vi "import ODB.vi"(0 "Dongle Fitted event Refnum in":T2, 2 "Programming Data":T4, 3 "APG Config":T3={"IPF Folder"=path "", "Results Folder"=path "", "Trace Folder"=path "", "a3DiCAD"={"Plot Spacing"=0.0, "TCF"=enum."STANDARD", "LeadLimit"=0, "a3DiCADDebug"=FALSE, "ODB"={"PrimePartNumber"=[], "SecondPartNumber"=[], "Height"={"PRP_CMP"="", "HEIGHT"=""}, "Units"={"PRP_CMP"="", "UNITS"=""}}, "PasteHeight"=0.0, "Inspection Performance"=TRUE}, "a3DiCADcfg"=path "", "Board Library"={"Board Library file"=path "", "Board library model folder"=path "", "Not Fittted/Fitted Components"=path "", "Panel Picture File"=path "", "Components"=enum."Fitted"}, "Site Library"={"Site Library file"=path "", "Site library model folder"=path ""}, "System Library"={"System Library file"=path "", "System library model folder"=path ""}, "ODB++ file"=path "", "Side ID Alias"={"Top"="", "Bottom"=""}}, 4 "Data":T10, 5 "error in":errorcluster, 6 "Edit VI":refnum<vi>, 7 "FP ctrl references":T1) -> (14 "Programming Data out":T4, 16 "Data out":T10, 17 "Dongle fitted":bool, 18 "APG Config":T3={"IPF Folder"=path "", "Results Folder"=path "", "Trace Folder"=path "", "a3DiCAD"={"Plot Spacing"=0.0, "TCF"=enum."STANDARD", "LeadLimit"=0, "a3DiCADDebug"=FALSE, "ODB"={"PrimePartNumber"=[], "SecondPartNumber"=[], "Height"={"PRP_CMP"="", "HEIGHT"=""}, "Units"={"PRP_CMP"="", "UNITS"=""}}, "PasteHeight"=0.0, "Inspection Performance"=TRUE}, "a3DiCADcfg"=path "", "Board Library"={"Board Library file"=path "", "Board library model folder"=path "", "Not Fittted/Fitted Components"=path "", "Panel Picture File"=path "", "Components"=enum."Fitted"}, "Site Library"={"Site Library file"=path "", "Site library model folder"=path ""}, "System Library"={"System Library file"=path "", "System library model folder"=path ""}, "ODB++ file"=path "", "Side ID Alias"={"Top"="", "Bottom"=""}}, 19 "error out":errorcluster)   [LabVIEW 2013, in "Manipulate IPF.lvlib"]
uses:
  Manipulate IPF.lvlib
  type_def/files.ctl
  3013/code/Modules/Inspection/Data/Panel_class/type_def/Config File data.ctl
  3013/code/Modules/Inspection/type_def/Pos and Rot.ctl
  3013/code/Modules/Inspection/Data/PCB_class/type_def/PCB Params.ctl
  3013/code/Modules/Inspection/Data/Panel_class/type_def/BarCode Params.ctl
  3013/code/Modules/Barcode Reader/type_def/id.ctl
  Settings/type_def/APG Config.ctl
  3013/code/Modules/GUI/GUI_5/subPanels/edit/type_def/data.ctl
  3013/code/Modules/Configuration/type_def/Scan Params.ctl
  3013/code/Modules/Configuration/type_def/Profile Resolution.ctl
  3013/code/Modules/Preprocess Data/type_def/direction.ctl
  3013/code/Modules/Inspection/Data/Panel_class/type_def/inspection data.ctl
  3013/code/Modules/Inspection/type_def/Range Limits.ctl
  type_def/Dongle fitted event refnum.ctl
  type_def/Import ODB state.ctl
  3013/code/Modules/Scanner/Robot/type_def/robot scan params DBL.ctl
  3013/code/Modules/Scanner/Robot/type_def/point DBL.ctl
  type_def/Picture FGV commands.ctl
  Pack Data/type_def/file types.ctl
  type_def/IPF cmd.ctl
  <userlib>/_OpenG.lib/file/file.llb/File Exists - Scalar__ogtk.vi
  <userlib>/_OpenG.lib/file/file.llb/Convert File Extension (Path)__ogtk.vi
  <vilib>/Utility/cursorutil.llb/Set Cursor (Icon Pict).vi
  Settings/Globals/apg_cfg_global.vi
  Conversion/conversion.lvlib
  3013/code/Modules/Configuration/Config.lvlib
  3013/code/Modules/Barcode Reader/Barcode Reader.lvlib
  3013/code/Modules/Inspection/Data/Panel_class/Panel.lvclass
  3013/code/Modules/Inspection/Inspection.lvlib
  3013/code/Modules/Inspection/Data/PCB_class/PCB.lvclass
  3013/code/Modules/Preprocess Data/PreProcess.lvlib
  3013/code/Modules/Scanner/Robot/Robot.lvlib
  3013/code/Modules/GUI/GUI_5/subPanels/edit/edit.lvlib
  Pack Data/Pack Files.lvlib
  Update TCF/TCF update.lvlib
  a3Di APG.lvlib
  Settings/APG_settings.lvlib
  Mike/APG_mike a3Di.lvlib
  Gerber import/Gerber import.lvlib
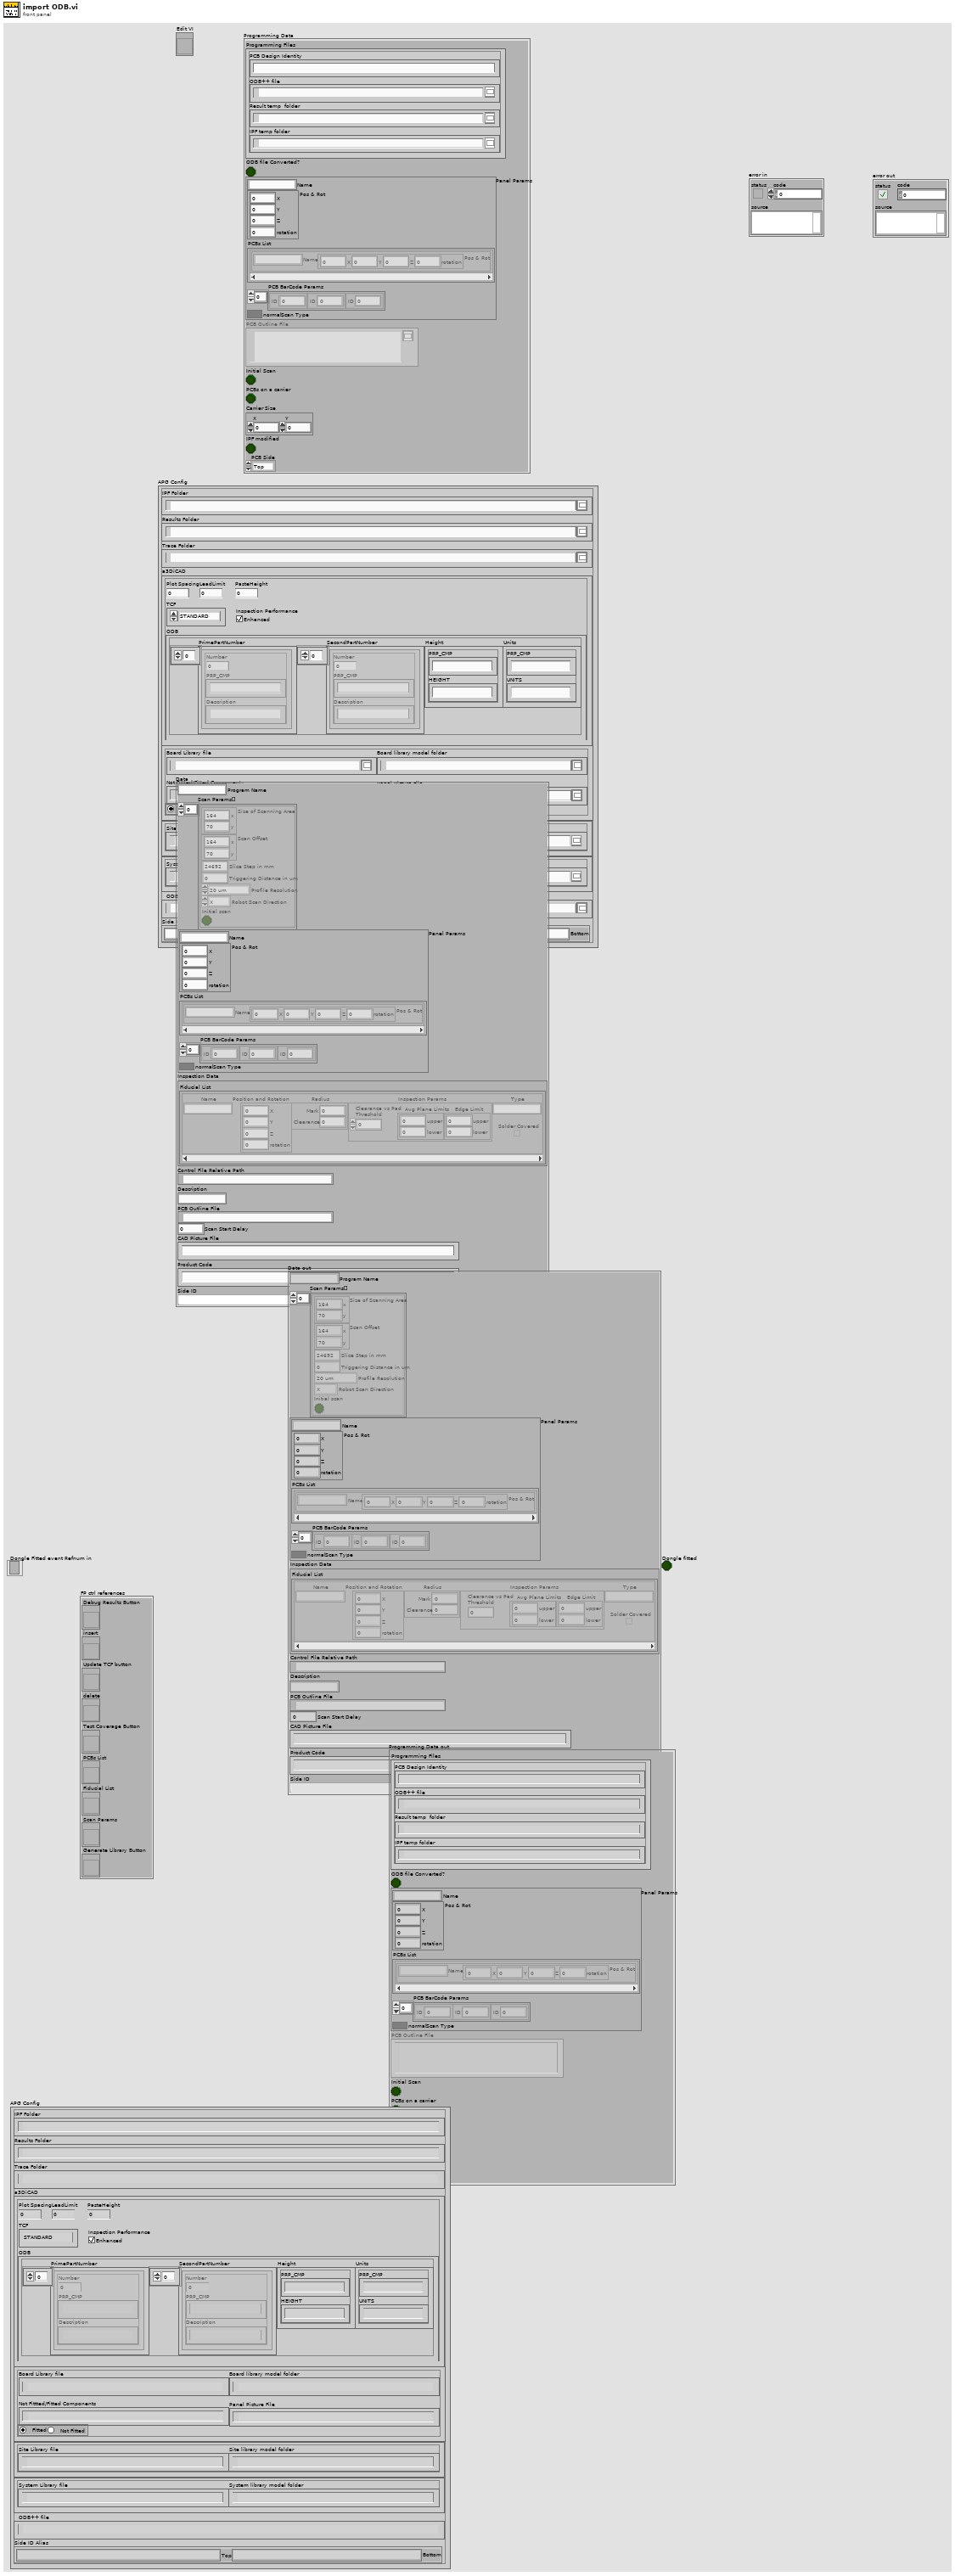
[diagram p1: front panel]
types:
  T1 = cluster{"Debug Results Button":refnum<vi>, "insert":refnum<vi>, "Update TCF button":refnum<vi>, "delete":refnum<vi>, "Test Coverage Button":refnum<vi>, "PCBs List":refnum<vi>, "Fiducial List":refnum<vi>, "Scan Params":refnum<vi>, "Generate Library Button":refnum<vi>}
  T2 = typedef "Dongle fitted event refnum.ctl" = refnum<event-registration>
  T3 = typedef "APG_settings.lvlib/APG Config.ctl" = cluster{"IPF Folder":path, "Results Folder":path, "Trace Folder":path, "a3DiCAD":cluster{"Plot Spacing":dbl, "TCF":enum16{"STANDARD", "PASTE", "LEAD"}, "LeadLimit":u32, "a3DiCADDebug":bool, "ODB":cluster{"PrimePartNumber":cluster{"Number":u32, "PRP_CMP":string, "Description":string}[], "SecondPartNumber":cluster{"Number":u32, "PRP_CMP":string, "Description":string}[], "Height":cluster{"PRP_CMP":string, "HEIGHT":string}, "Units":cluster{"PRP_CMP":string, "UNITS":string}}, "PasteHeight":dbl, "Inspection Performance":bool}, "a3DiCADcfg":path, "Board Library":cluster{"Board Library file":path, "Board library model folder":path, "Not Fittted/Fitted Components":path, "Panel Picture File":path, "Components":enum32{"Fitted", "Not Fitted "}}, "Site Library":cluster{"Site Library file":path, "Site library model folder":path}, "System Library":cluster{"System Library file":path, "System library model folder":path}, "ODB++ file":path, "Side ID Alias":cluster{"Top":string, "Bottom":string}}
  T4 = typedef "a3Di APG.lvlib/files.ctl" = cluster{"Programming Files":cluster{"PCB Design Identity":string, "ODB++ file":path, "Result temp  folder":path, "IPF temp folder":path}, "ODB file Converted?":bool, "Panel Params":T5, "PCB Outline File":path, "Initial Scan":bool, "PCBs on a carrier":bool, "Carrier Size":cluster{"X":dbl, "Y":dbl}, "IPF modified":bool, "PCB Side":enum16{"Top", "Bottom"}}
  T5 = typedef "Inspection.lvlib/Panel.lvclass/Config File data.ctl" = cluster{"Name":string, "Pos & Rot":T6, "PCBs List":cluster{"PCB Params":T7}[], "PCB BarCode Params":T8[], "Scan Type":bool}
  T6 = typedef "Inspection.lvlib/Pos and Rot.ctl" = cluster{"X":dbl, "Y":dbl, "Z":dbl, "rotation":dbl}
  T7 = typedef "Inspection.lvlib/PCB.lvclass/PCB Params.ctl" = cluster{"Name":string, "Pos & Rot":T6}
  T8 = typedef "Inspection.lvlib/Panel.lvclass/BarCode Params.ctl" = cluster{"ID":T9}
  T9 = typedef "Barcode Reader.lvlib/id.ctl" = u8
  T10 = typedef "GUI.lvlib/subPanel.lvlib/edit.lvlib/data.ctl" = cluster{"Program Name":string, "Scan Params[]":T11[], "Panel Params":T5, "Inspection Data":T14, "Control File Relative Path":path, "Description":string, "PCB Outline File":path, "Scan Start Delay":dbl, "CAD Picture File":string, "Product Code":string, "Side ID":string}
  T11 = typedef "Config.lvlib/Scan Params.ctl" = cluster{"Size of Scanning Area":cluster{"x":dbl, "y":dbl}, "Scan Offset":cluster{"x":dbl, "y":dbl}, "Slice Step in mm":dbl, "Triggering Distance in mm":dbl, "Triggering Distance in um":dbl, "Profile Resolution":T12, "Version":string, "Robot Scan Direction":T13, "Initial scan":bool}
  T12 = typedef "Config.lvlib/Profile Resolution.ctl" = enum8{"20 um", "40 um"}
  T13 = typedef "PreProcess.lvlib/direction.ctl" = enum8{"X", "Y"}
  T14 = typedef "Inspection.lvlib/Panel.lvclass/inspection data.ctl" = cluster{"Fiducial List":cluster{"Name":string, "Position and Rotation":T6, "Radius":cluster{"Mark":dbl, "Clearance":dbl}, "Inspection Params":cluster{"Clearance vs Pad\nThreshold":dbl, "Avg Plane Limits":T15, "Edge Limit":T15}, "Type":string, "Solder Covered":bool}[]}
  T15 = typedef "Inspection.lvlib/Range Limits.ctl" = cluster{"upper":sgl, "lower":sgl}
  T16 = typedef "Manipulate IPF.lvlib/Import ODB state.ctl" = enum16{"Select format", "Select ODB++", "Extract ODB++", "Extract Gerber", "Select PCBs", "Scan area", "Select Fiducials", "Update TCF, save Files", "Cancel", "Exit", "Update CAD Picture"}
  T17 = typedef "Robot.lvlib/robot scan params DBL.ctl" = cluster{"Zero":T18, "Zero Speed":T18, "Distance":T18, "Speed":T18, "# of Slices":dbl, "Trigg Distance":dbl, "Robot Scan Direction":T13, "Next":cluster{"Next Zero":T18, "Next Robot Scan Direction":T13}}
  T18 = typedef "Robot.lvlib/point DBL.ctl" = cluster{"X":dbl, "Y":dbl}
  T19 = cluster{"Programming Files":cluster{"PCB Design Identity":string, "ODB++ file":path, "Result  folder":path, "Tar file":path}, "ODB file Converted?":bool, "Inspection Setup Data":cluster{"Inspection Program  file ":path, "PCB Scanning Area":cluster{"X":dbl, " Y":dbl}, "PCB Offset":cluster{" X":dbl, " Y":dbl}, "Scanning area  bot left and top right":cluster{"X":dbl, "Y":dbl}[], "Fiducials from scan":cluster{"Fiducial Name":string, "Fiducial co-ordinate":cluster{"X":dbl, "Y":dbl}}[], "TCF  file ":path, "Robot Scan Params DBL":T17, "Scan offset adjustment":cluster{"X":dbl, " Y":dbl}}, "Panel Params":T5, "PCB Outline File":path, "Inspection setup completed":bool, "PCB Layer scanned":enum16{"Bottom PCB Layer", "Top PCB Layer"}, "PCBs on a carrier":bool, "Carrier Size":cluster{"X":dbl, "Y":dbl}}
  T20 = typedef "Manipulate IPF.lvlib/Picture FGV commands.ctl" = enum16{"No Action", "Set Update Picture", "Set Delete Picture", "Get Picture action"}
  T21 = typedef "Pack Files.lvlib/file types.ctl" = enum16{"ODB", "TCF", "CAD Outline", "Config", "Inspection Prog", "a3Di-bin", "Results", "CAD Labels", "CAD Pads", "calScan_fid", "calScan_cal-tab", "PCB_SerialNumber", "CAD_Assembly", "Version", "Old Results", "CAD Picture", "Old TCF"}
  T22 = typedef "Manipulate IPF.lvlib/IPF cmd.ctl" = enum16{"New IPF", "Edit IPF", "Copy IPF", "Rename IPF", "Delete IPF", "Reload IPF", "Load all IPF"}
  T23 = enum16{"Left Button", "Center Button", "Right Button", "Window Close"}
  T24 = typedef "GUI.lvlib/subPanel.lvlib/edit.lvlib/GUI Panel & PCB params.ctl" = cluster{"Panel Params":T25, "PCBs List":T26}
  T25 = typedef "GUI.lvlib/subPanel.lvlib/edit.lvlib/GUI Panel Params.ctl" = cluster{"Name":string, "Pos & Rot":T6}
  T26 = typedef "GUI.lvlib/subPanel.lvlib/edit.lvlib/GUI PCB List.ctl" = cluster{"PCB Params":T7, "Barcode\nReader":cluster{"ID":T9}, "insert":bool, "delete":bool}[]
  T27 = cluster{"Scanning Area X in mm":dbl, "Scanning Area Y in mm":dbl}
  T28 = typedef "GUI.lvlib/subPanel.lvlib/edit.lvlib/GUI Fiducial List.ctl" = cluster{"Fiducial":cluster{"Name":string, "Pos & Rot":T6, "Radius":cluster{"Mark":dbl, "Clearance":dbl}, "Inspection Params":cluster{"Clearance vs\nPad Threshold":dbl, "Avg Plane Limits":T15, "Edge Limit":T15}, "Type":string, "Solder Covered":bool}, "insert":bool, "delete":bool}[]
  T29 = enum8{"Enabled", "Disabled", "Disabled and Grayed Out"}
  T30 = cluster{"APG":cluster{"APG SIN":string, "APG version":string}, "Installed Programs":cluster{"task name":string, "task version":string}[]}
  T31 = cluster{"task name":string, "task version":string}[]
  T32 = cluster{"Program":enum16{"APG", "Inspection Station"}, "APG":cluster{"APG SIN":string, "APG version":string}, "Installed Programs":cluster{"task name":string, "task version":string}[]}
  T33 = typedef "Manipulate IPF.lvlib/Picture FGV actions.ctl" = enum16{"No Action", "Update Picture", "Delete Picture"}
  T34 = cluster{"Name":string, "Position and Rotation":T6, "Radius":cluster{"Mark":dbl, "Clearance":dbl}, "Inspection Params":cluster{"Clearance vs Pad\nThreshold":dbl, "Avg Plane Limits":T15, "Edge Limit":T15}, "Type":string, "Solder Covered":bool}[]
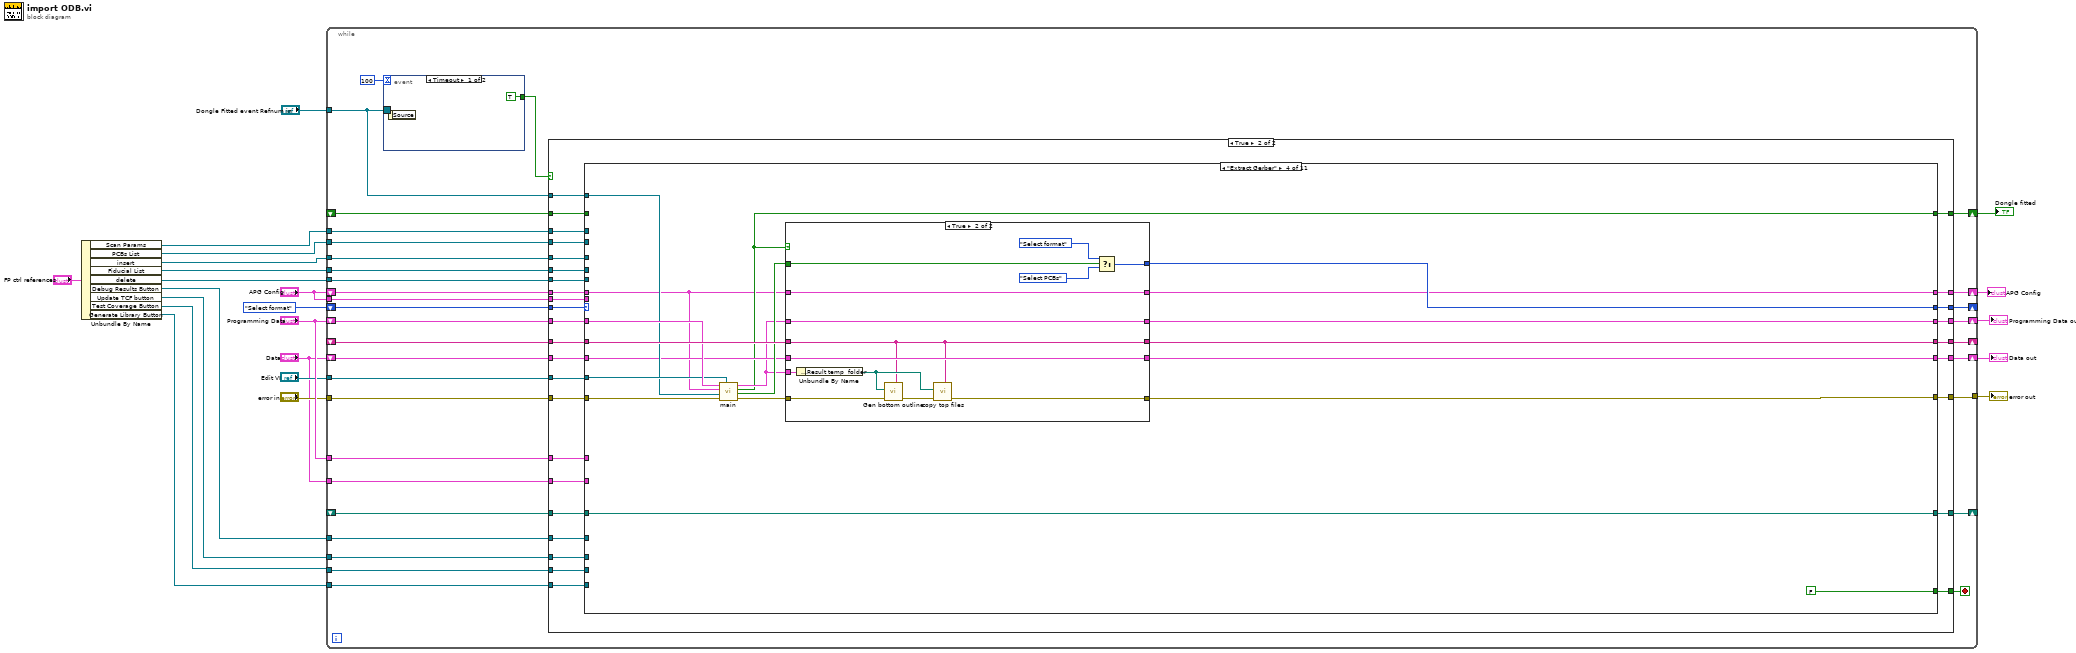
[diagram p0: block diagram]
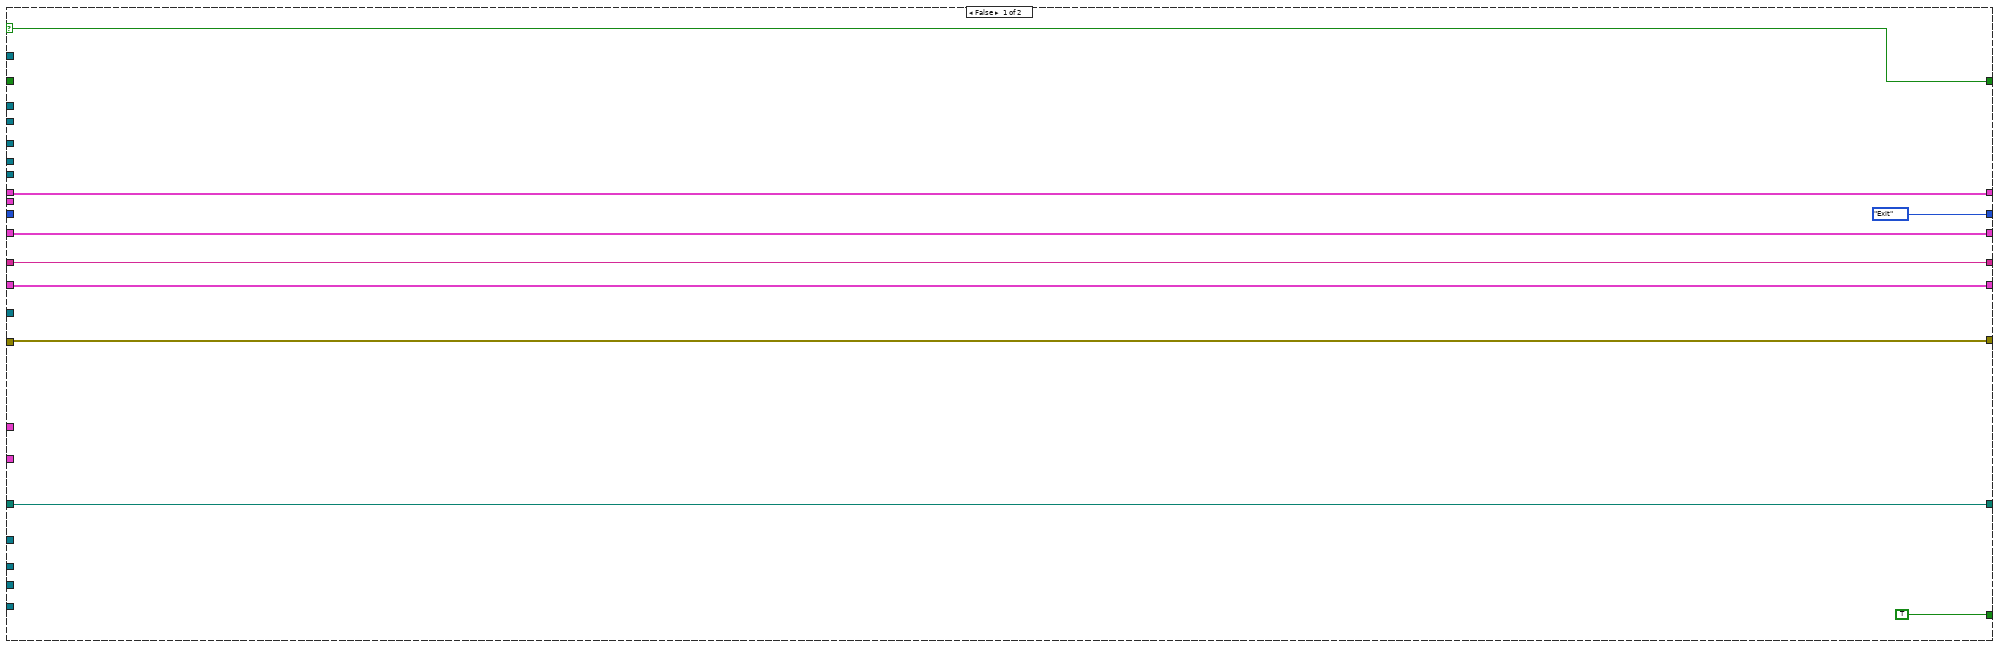
[diagram p2: hidden frame]
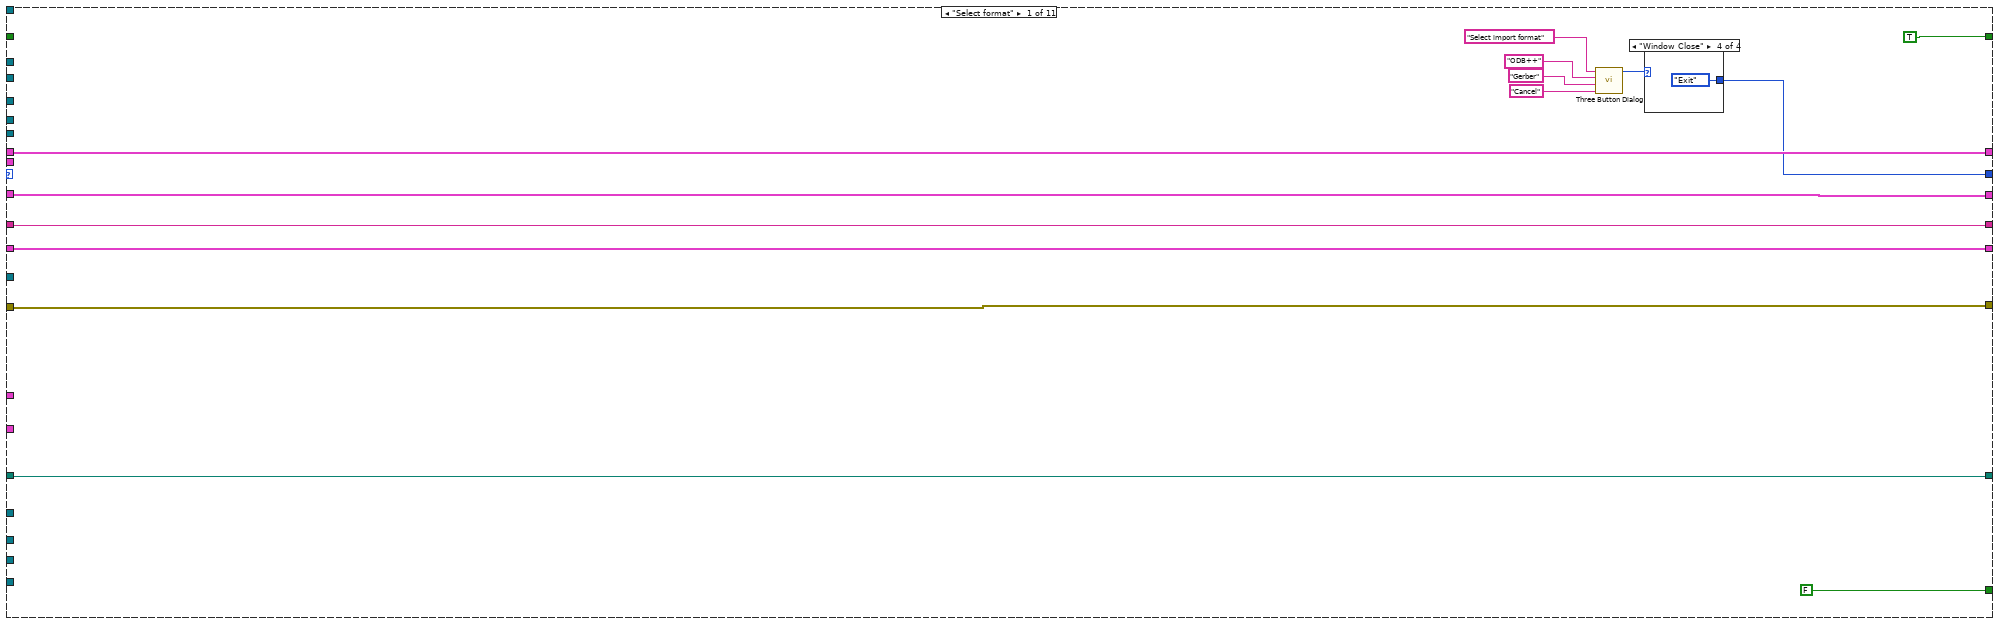
[diagram p3: hidden frame]
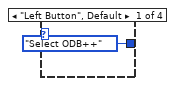
[diagram p4: hidden frame]
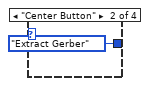
[diagram p5: hidden frame]
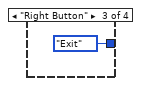
[diagram p6: hidden frame]
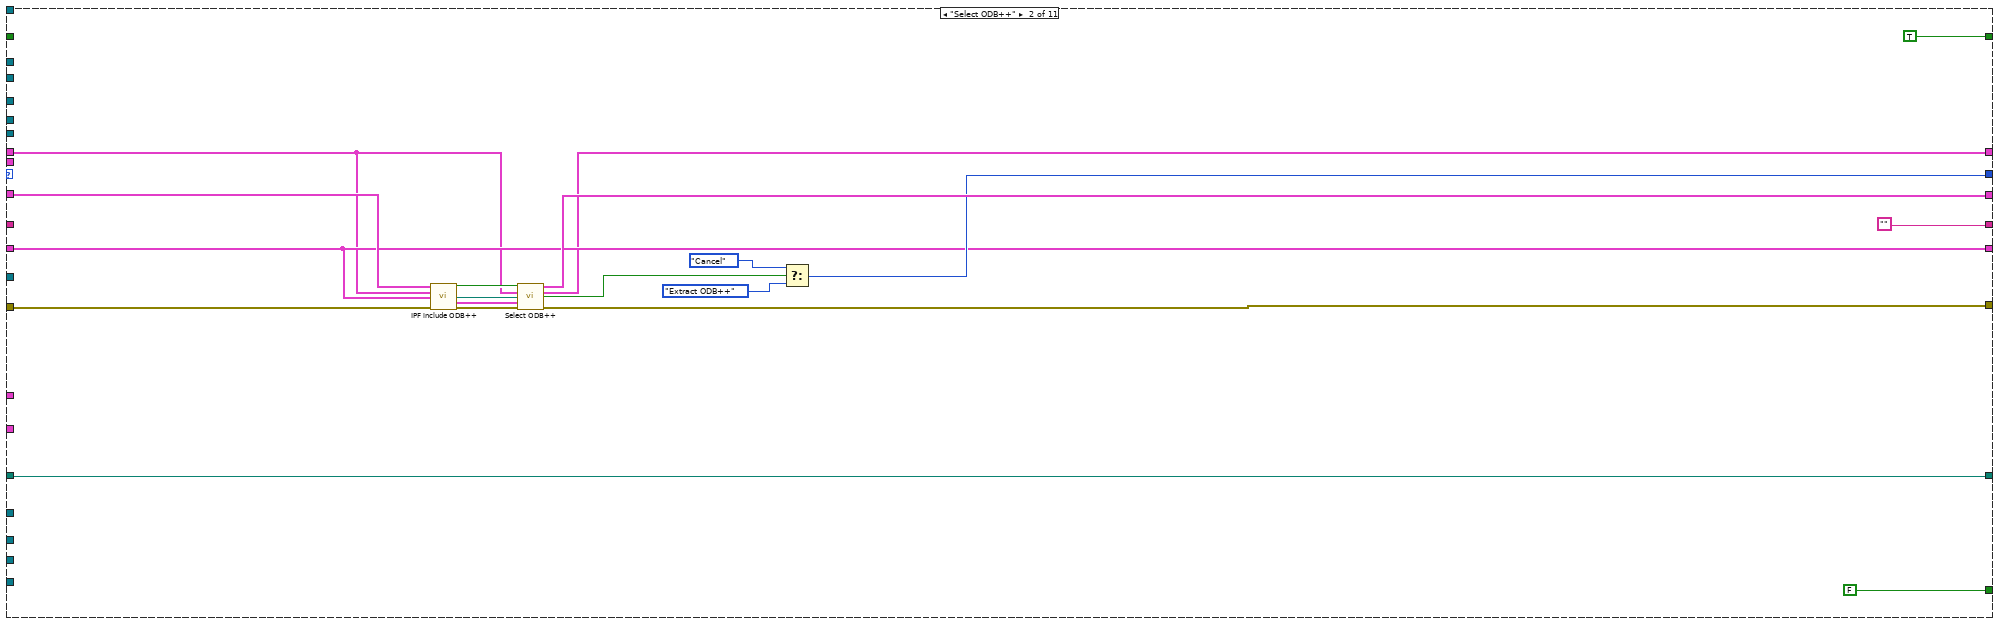
[diagram p7: hidden frame]
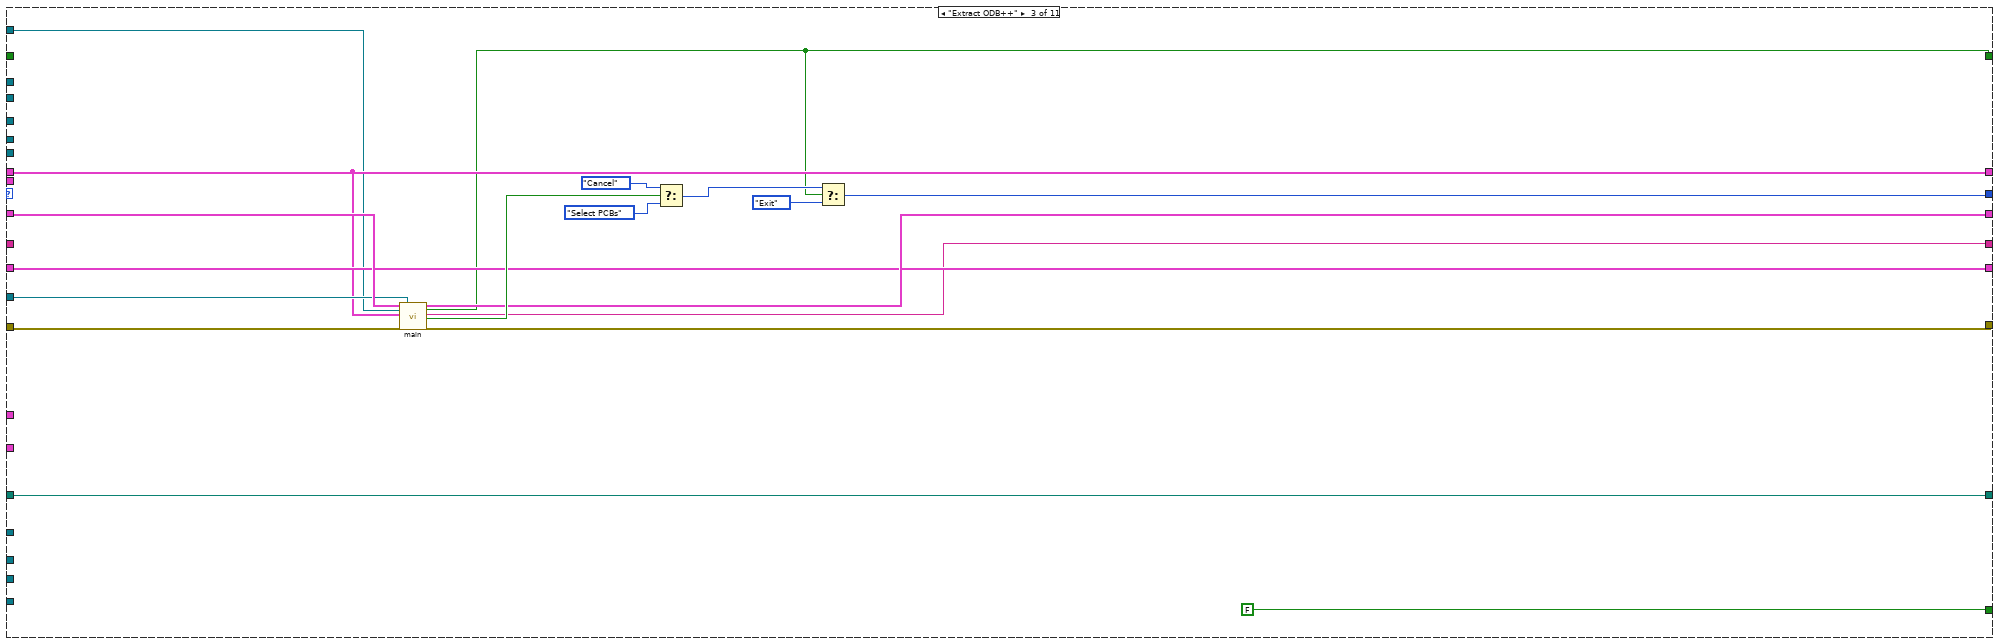
[diagram p8: hidden frame]
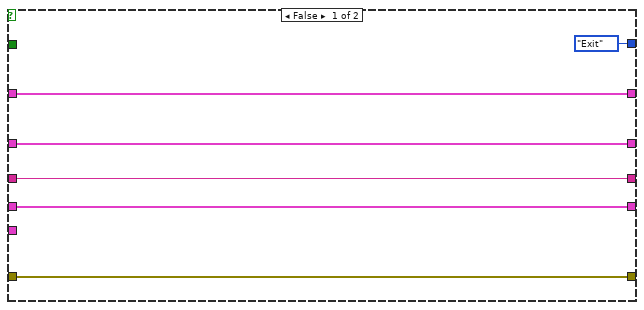
[diagram p9: hidden frame]
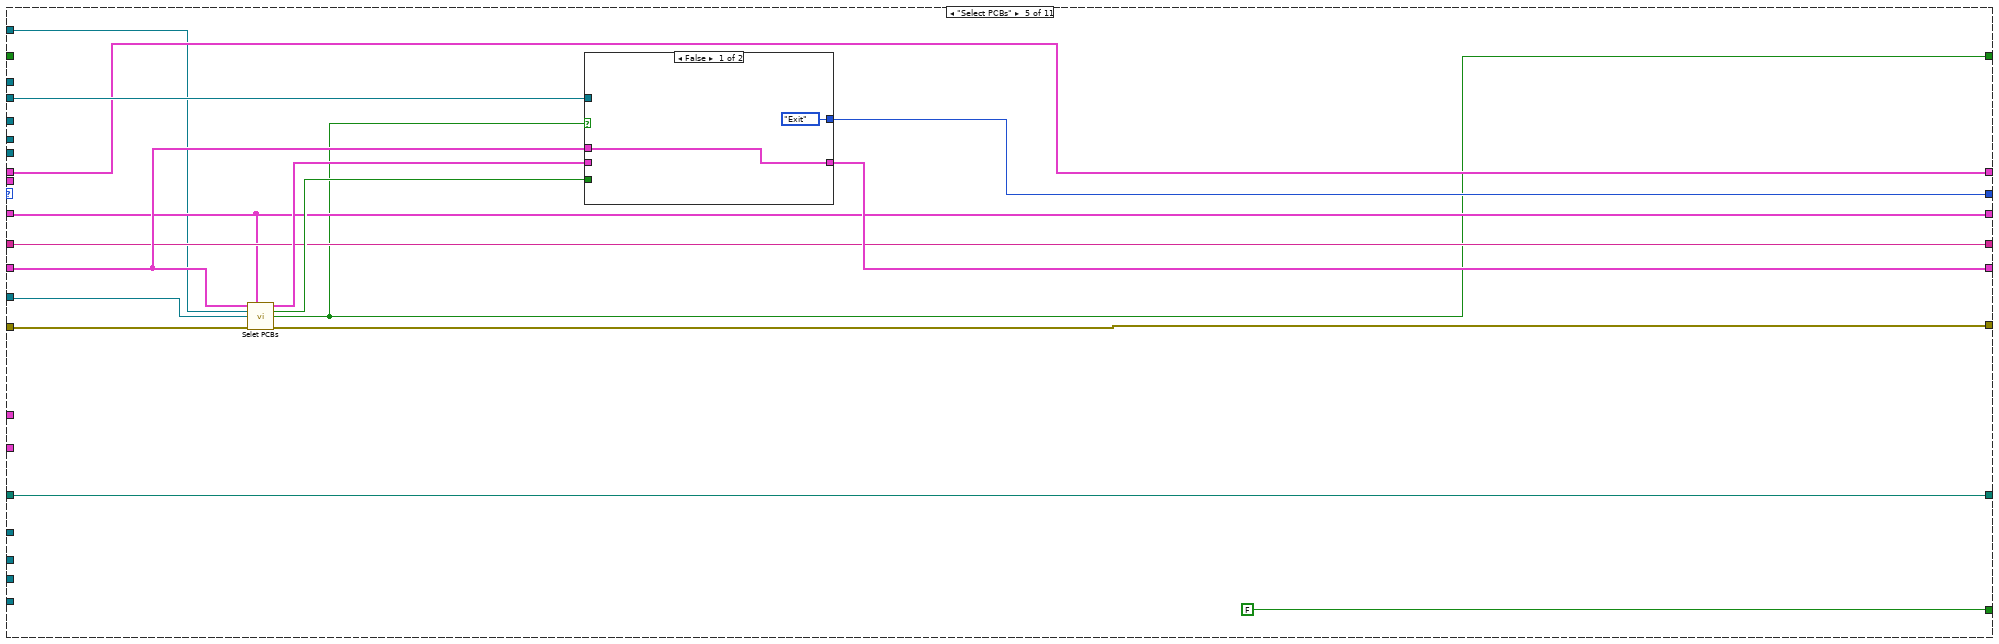
[diagram p10: hidden frame]
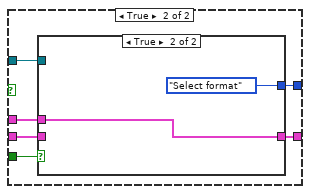
[diagram p11: hidden frame]
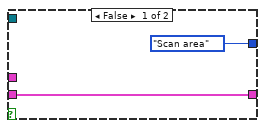
[diagram p12: hidden frame]
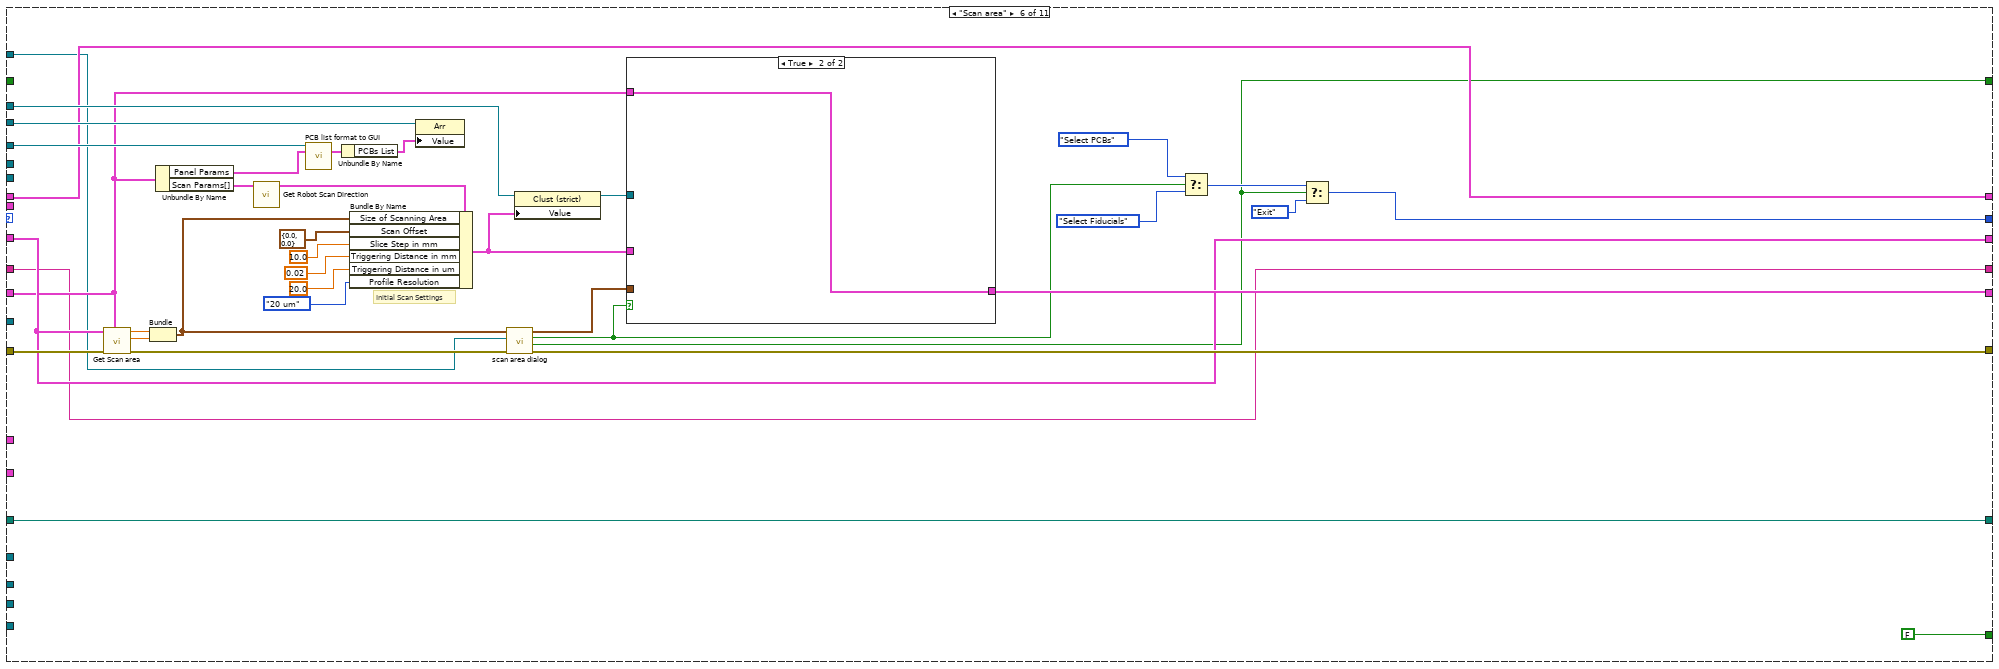
[diagram p13: hidden frame]
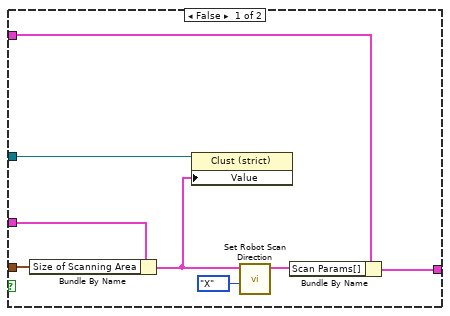
[diagram p14: hidden frame]
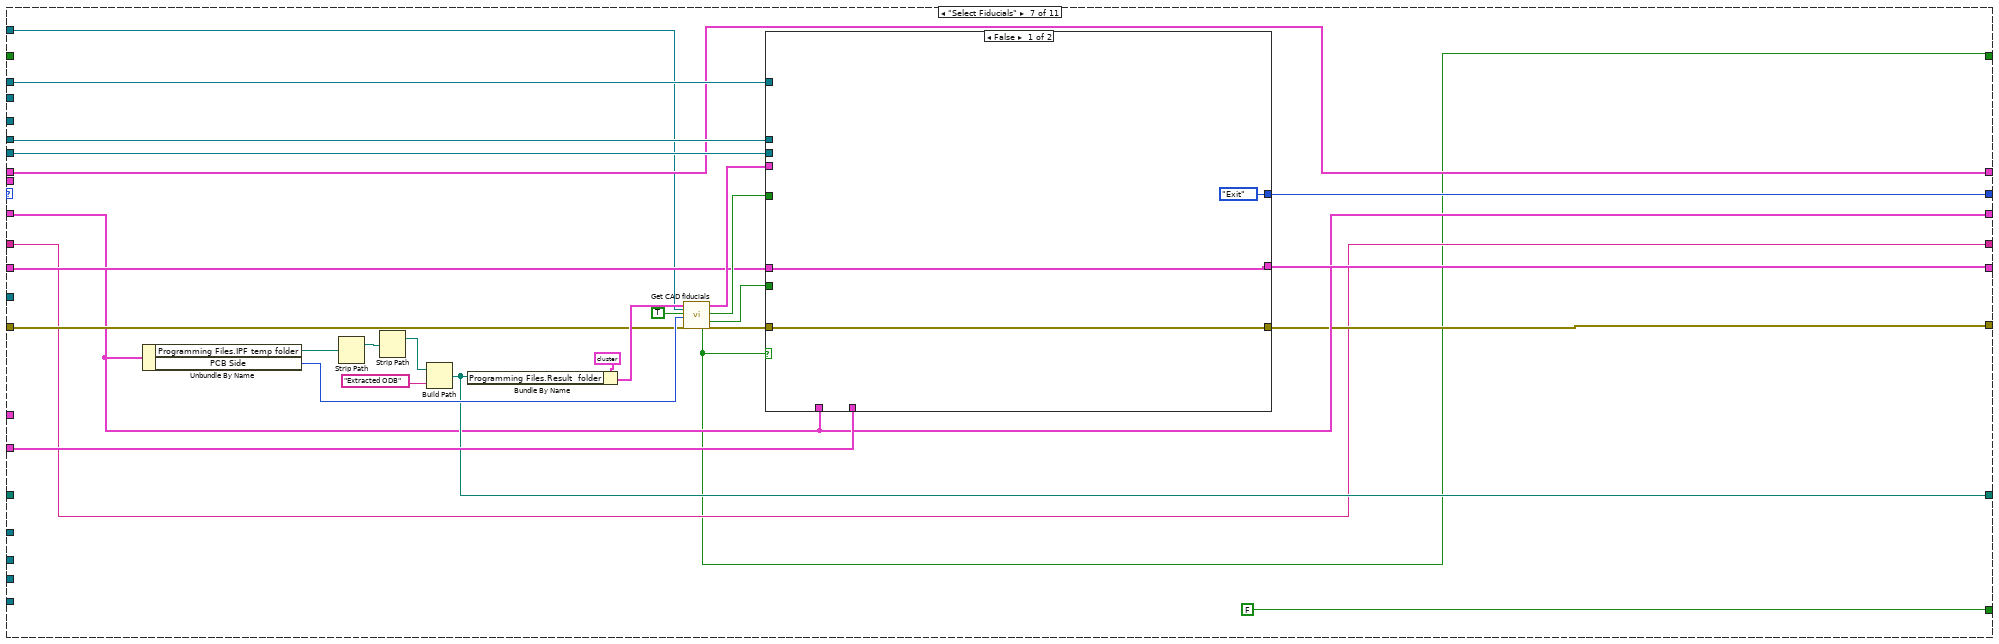
[diagram p15: hidden frame]
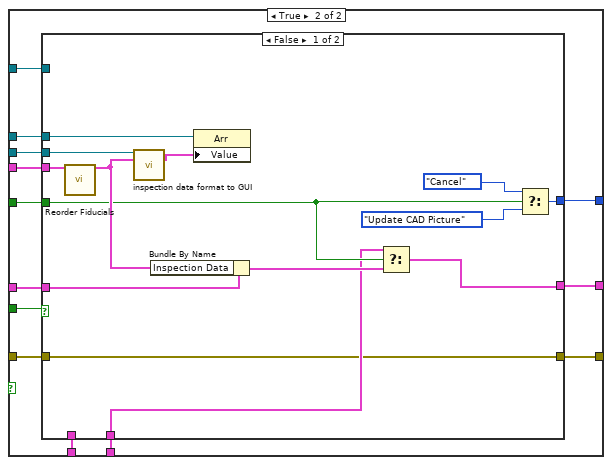
[diagram p16: hidden frame]
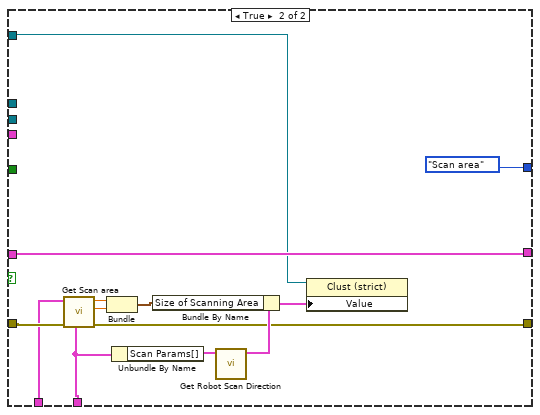
[diagram p17: hidden frame]
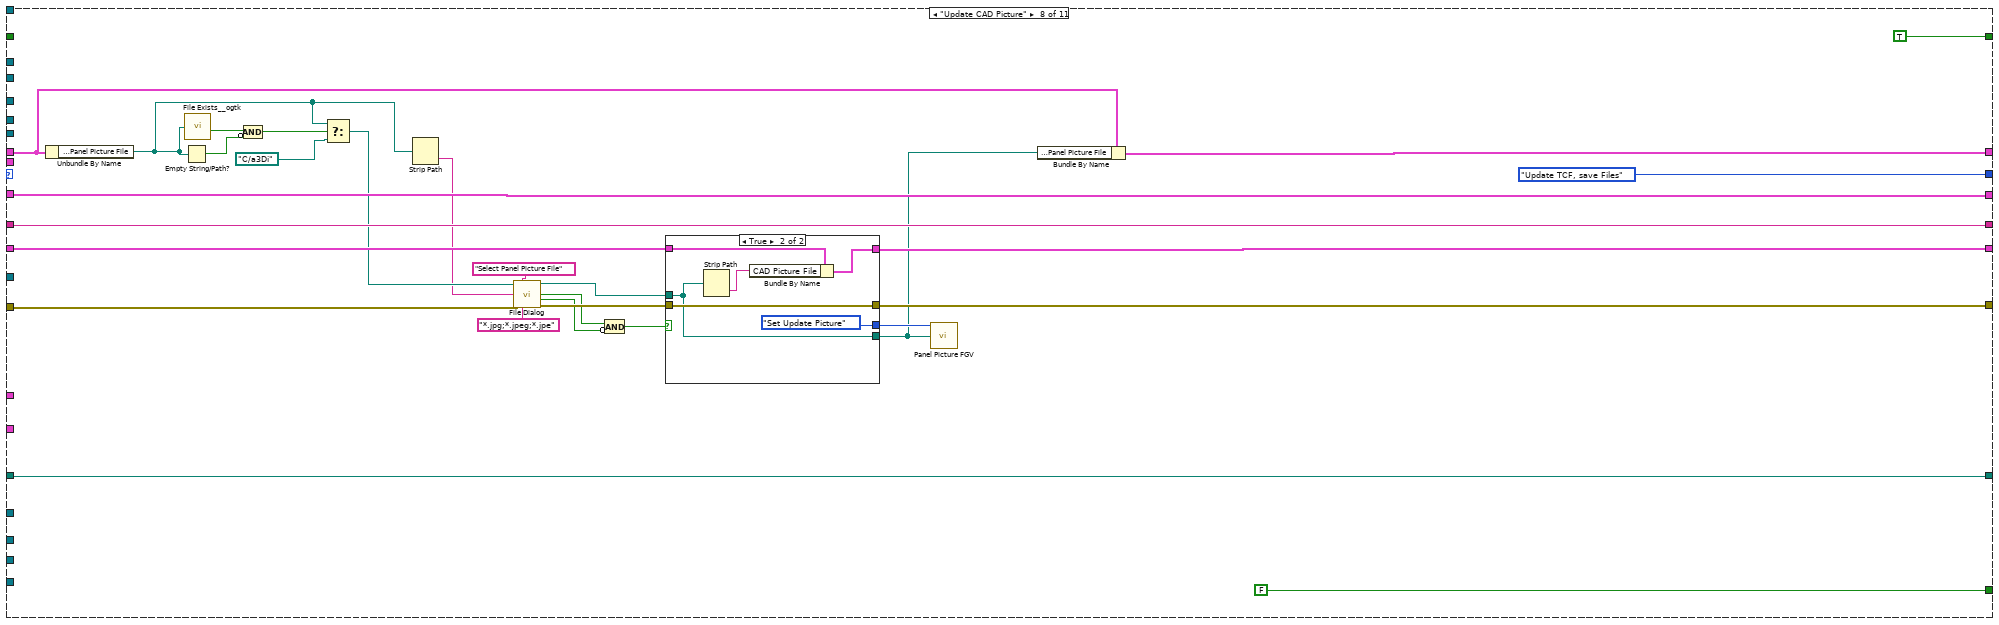
[diagram p18: hidden frame]
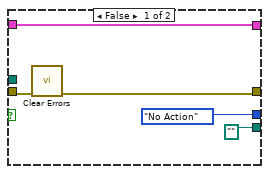
[diagram p19: hidden frame]
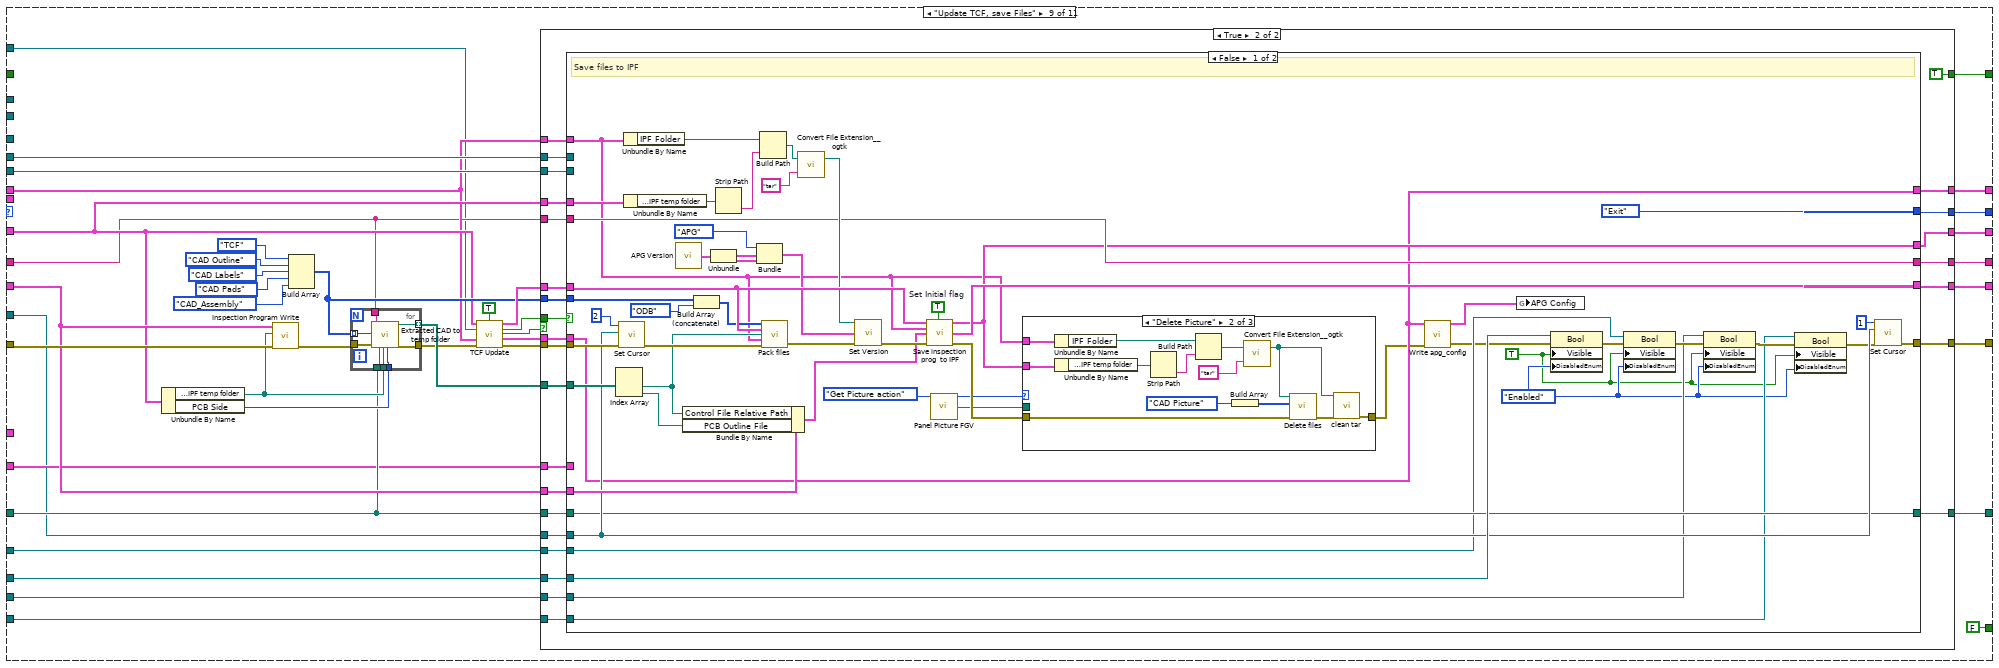
[diagram p20: hidden frame]
diagram:
  n1 = Unbundle By Name("FP ctrl references") -> ("Scan Params"=w9:refnum<vi>, "PCBs List"=w8:refnum<vi>, "insert"=w10:refnum<vi>, "Fiducial List"=w7:refnum<vi>, "delete"=w6:refnum<vi>, "Debug Results Button"=w5:refnum<vi>, "Update TCF button"=w4:refnum<vi>, "Test Coverage Button"=w3:refnum<vi>, "Generate Library Button"=w2:refnum<vi>)
  n2 = while {
    tunnel: "error in" -> [w54]
    tunnel: [w33] -> w20
    shift-right: [w51] -> w18
    shift-left: "Programming Data" -> [w50]
    shift-right: [w49] -> _
    shift-left: Import_ODB_state."Select format" -> [w55]
    tunnel: "Edit VI" -> [w48]
    shift-right: [w29] -> w19
    shift-left: "Data" -> [w47]
    tunnel: w9 -> [w46]
    tunnel: w8 -> [w45]
    tunnel: w10 -> [w44]
    tunnel: w7 -> [w43]
    tunnel: w6 -> [w42]
    tunnel: "Data" -> [w41]
    tunnel: "Programming Data" -> [w40]
    shift-right: [w39] -> _
    shift-left: _ -> [w38]
    tunnel: w4 -> [w37]
    tunnel: w5 -> [w36]
    shift-right: [w34] -> _
    shift-left: _ -> [w35]
    shift-right: [w32] -> w14
    shift-left: "APG Config" -> [w53]
    tunnel: "APG Config" -> [w31]
    tunnel: w3 -> [w30]
    tunnel: w2 -> [w28]
    tunnel: "Dongle Fitted event Refnum in" -> [w25]
    shift-right: [w24] -> w1
    shift-left: _ -> [w23]
    stop <- w52 stop-if-true
    n3 = event shown="[0] Timeout" {
      selector: w25 -> [_ _]
      dyn-events: _ -> [_ _]
      timeout: 100 -> [_ _]
      tunnel: [TRUE FALSE] -> w26
      event Timeout {
        n4 = event-data() -> ()  [unwired: 1 in, 1 out]
      }
      event User Event {
        n5 = event-data() -> ()  [unwired: 1 in, 1 out]
      }
    }
    n6 = case shown="True" w26 {
      selector: w26 -> [w56 _]
      tunnel: w55 -> [_ w95]
      tunnel: w54 -> [w58 w94]
      tunnel: w53 -> [w62 w93]
      tunnel: [TRUE w92] -> w52
      tunnel: [w61 w91] -> w51
      tunnel: w50 -> [w61 w90]
      tunnel: [Import_ODB_state."Exit" w89] -> w49
      tunnel: w48 -> [_ w88]
      tunnel: w47 -> [w59 w87]
      tunnel: w46 -> [_ w86]
      tunnel: w45 -> [_ w85]
      tunnel: w44 -> [_ w84]
      tunnel: w43 -> [_ w83]
      tunnel: w42 -> [_ w82]
      tunnel: w41 -> [_ w81]
      tunnel: w40 -> [_ w80]
      tunnel: [w57 w79] -> w39
      tunnel: w38 -> [w57 w78]
      tunnel: w37 -> [_ w77]
      tunnel: w36 -> [_ w76]
      tunnel: w35 -> [w60 w75]
      tunnel: [w60 w74] -> w34
      tunnel: [w58 w73] -> w33
      tunnel: [w62 w72] -> w32
      tunnel: w31 -> [_ w71]
      tunnel: w30 -> [_ w70]
      tunnel: [w59 w69] -> w29
      tunnel: w28 -> [_ w68]
      tunnel: w25 -> [_ w67]
      tunnel: [w56 w66] -> w24
      tunnel: w23 -> [_ w65]
      frame False {
      }
      frame True {
        n7 = case shown="\"Extract Gerber\"" w95 {
          tunnel: w94 -> [w108 w129 w150 w165 w202 w253 w273 w359 w409 w557 w569]
          tunnel: w93 -> [w102 w116 w138 w151 w191 w222 w265 w346 w384 w548 w570]
          tunnel: w90 -> [w103 w128 w149 w163 w193 w225 w269 w355 w386 _ w566]
          tunnel: [w103 w127 w144 w155 w193 w225 w269 w355 w390 w554 w565] -> w91
          tunnel: [FALSE FALSE FALSE FALSE FALSE FALSE FALSE FALSE FALSE FALSE TRUE] -> w92
          tunnel: [w97 w123 w134 w166 w199 w218 w282 Import_ODB_state."Update TCF, save Files" w394 Import_ODB_state."Exit" Import_ODB_state."Exit"] -> w89
          tunnel: w80 -> [_ _ _ _ _ _ _ _ _ w554 _]
          tunnel: w88 -> [_ _ w148 w162 w192 _ _ _ w381 _ _]
          tunnel: w87 -> [w105 w121 w143 w159 w198 w224 w272 w357 w402 _ w573]
          tunnel: w86 -> [_ _ _ _ _ w229 w268 _ _ _ _]
          tunnel: w85 -> [_ _ _ _ w195 w230 _ _ _ _ _]
          tunnel: w84 -> [_ _ _ _ _ w238 _ _ _ _ _]
          tunnel: w83 -> [_ _ _ _ _ _ w280 _ w388 _ _]
          tunnel: w82 -> [_ _ _ _ _ _ w279 _ w387 _ _]
          tunnel: w81 -> [_ _ _ _ _ _ w276 _ w389 w553 _]
          tunnel: [w106 w118 w140 w169 w203 w236 w274 w360 w392 w551 w572] -> w79
          tunnel: w78 -> [w106 w118 w140 w169 w203 w236 _ w360 w393 w551 w572]
          tunnel: w77 -> [_ _ _ _ _ _ _ _ w397 _ _]
          tunnel: w76 -> [_ _ _ _ _ _ _ _ w396 _ _]
          tunnel: w75 -> [w104 _ _ w168 w194 w223 w266 w354 w382 w550 w571]
          tunnel: [w104 "" w139 w157 w194 w223 w266 w354 w383 w550 w571] -> w74
          tunnel: [w108 w119 w141 w153 w201 w235 w267 w358 w399 w552 w568] -> w73
          tunnel: [w102 w115 w138 w154 w191 w222 w265 w345 w379 w549 w570] -> w72
          tunnel: w71 -> [_ _ _ _ _ _ _ _ _ w549 _]
          tunnel: w70 -> [_ _ _ _ _ _ _ _ w378 _ _]
          tunnel: [w105 w121 w143 w158 w196 w232 w277 w356 w398 w553 w573] -> w69
          tunnel: w68 -> [_ _ _ _ _ _ _ _ w376 _ _]
          tunnel: w67 -> [_ _ w137 w160 w190 w221 w264 _ w375 _ _]
          tunnel: [TRUE ("Dongle fitted") TRUE ("Dongle fitted") w133 w152 w189 w217 w263 TRUE ("Dongle fitted") w373 TRUE ("Dongle fitted") w564] -> w66
          tunnel: w65 -> [_ _ _ _ _ _ _ _ _ _ w564]
          frame "Select format" {
            n8 = call <vilib>:"Three Button Dialog.vi"("Right Button Text (\"Cancel\")"="Cancel" ("Right Button Text (\"Cancel\")"), "Center Button Text (\"No\")"="Gerber" ("F button name (\"Cancel\")"), "Left Button Text (\"Yes\")"="ODB++" ("T button name (\"OK\")"), "message"="Select import format") -> ("Which Button?"=w98:T23)  [unwired: 7 in]
            n9 = case shown="\"Window Close\"" w98 {
              tunnel: [Import_ODB_state."Select ODB++" Import_ODB_state."Extract Gerber" Import_ODB_state."Exit" Import_ODB_state."Exit"] -> w97
              frame "Left Button", Default {
              }
              frame "Center Button" {
              }
              frame "Right Button" {
              }
              frame "Window Close" {
              }
            }
          }
          frame "Select ODB++" {
            n10 = call "IPF include ODB++.vi"("Programming Data"=w128, "APG Config"=w116, "Data"=w121, "error in"=w129) -> ("IPF include ODB++"=w130:bool, "ODB++ file"=w131:path, "Programming Data out"=w120:T4, "error out"=w132:errorcluster)  [unwired: 8 in]
            n11 = call "Select ODB++.vi"("IPF include ODB++"=w130, "APG Config"=w116, "ODB++ file"=w131, "Programming Data"=w120, "error in"=w132) -> ("Programming data"=w127:T4, "APG Config"=w115:T3, "cancelled"=w125:bool, "error out"=w119:errorcluster)  [unwired: 7 in]
            n12 = Select(t=Import_ODB_state."Cancel", s=w125, f=Import_ODB_state."Extract ODB++") -> (s? t:f=w123:T16)
          }
          frame "Extract ODB++" {
            n13 = call "main.vi"("Programming Data In"=w149, "Dongle Fitted event Refnum in"=w137, "APG Config"=w138, "error in"=w150, "Edit VI"=w148) -> ("Programming Data out"=w144:T4, "Dongle fitted"=w133:bool, "Assembly"=w139:string, "Extraction Failed"=w147:bool, "error out"=w141:errorcluster)  [unwired: 10 in]
            n14 = Select(t=Import_ODB_state."Cancel", s=w147, f=Import_ODB_state."Select PCBs") -> (s? t:f=w136:T16)
            n15 = Select(t=w136, s=w133, f=Import_ODB_state."Exit") -> (s? t:f=w134:T16)
          }
          frame "Extract Gerber" {
            n16 = call "main.vi"("Edit VI"=w162, "error in"=w165, "Dongle Fitted event Refnum in"=w160, "APG Config"=w151, "Programming Data In"=w163) -> ("error out"=w164:errorcluster, "Conversion Cancled"=w161:bool, "Dongle fitted"=w152:bool, "Programming Data Out"=w156:T4)  [unwired: 3 in]
            n17 = case shown="True" w152 {
              tunnel: w168 -> [w172 w178]
              tunnel: [Import_ODB_state."Exit" w183] -> w166
              tunnel: w164 -> [w174 w182]
              tunnel: w156 -> [_ w181]
              tunnel: w161 -> [_ w180]
              tunnel: w159 -> [w173 w179]
              tunnel: [w173 w179] -> w158
              tunnel: [w172 w178] -> w157
              tunnel: w156 -> [w171 w177]
              tunnel: [w171 w177] -> w155
              tunnel: w151 -> [w170 w176]
              tunnel: [w170 w176] -> w154
              tunnel: [w174 w187] -> w153
              frame False {
              }
              frame True {
                n18 = Unbundle By Name(w181) -> ("Programming Files.Result temp  folder"=w186:path)
                n19 = call "Gen bottom outline.vi"("Assembly"=w178, "error in (no error)"=w182, "results folder"=w186) -> ("error out"=w188:errorcluster)  [unwired: 6 in, 2 out]
                n20 = call "copy top files.vi"("Assembly"=w178, "error in (no error)"=w188, "results folder"=w186) -> ("error out"=w187:errorcluster)  [unwired: 7 in, 1 out]
                n21 = Select(t=Import_ODB_state."Select format", s=w180, f=Import_ODB_state."Select PCBs") -> (s? t:f=w183:T16)
              }
            }
          }
          frame "Select PCBs" {
            n22 = call "Selet PCBs.vi"("data in"=w198, "Programming Data"=w193, "Dongle Fitted event Refnum in"=w190, "Edit VI"=w192, "error in"=w202) -> ("data out"=w197:T10, "Back"=w200:bool, "Dongle fitted"=w189:bool, "error out"=w201:errorcluster)  [unwired: 7 in]
            n23 = case shown="False" w189 {
              tunnel: w200 -> [_ w212]
              tunnel: [Import_ODB_state."Exit" w211] -> w199
              tunnel: w198 -> [w205 w210]
              tunnel: w197 -> [_ w209]
              tunnel: [w205 w208] -> w196
              tunnel: w195 -> [_ w207]
              frame False {
              }
              frame True {
                n24 = case shown="True" w212 {
                  tunnel: [Import_ODB_state."Scan area" Import_ODB_state."Select format"] -> w211
                  tunnel: w210 -> [_ w215]
                  tunnel: w209 -> [w214 _]
                  tunnel: [w214 w215] -> w208
                  tunnel: w207 -> [_ _]
                  frame False {
                  }
                  frame True {
                  }
                }
              }
            }
          }
          frame "Scan area" {
            # "Initial Scan Settings"
            n25 = call "Get Scan area.vi"("Inspection data"=w224, "error in (no error)"=w253, "Programming Data"=w225) -> ("error out"=w243:errorcluster, "Panel size Y"=w251:dbl, "Panel Size X"=w252:dbl)  [unwired: 6 in]
            n26 = Bundle("Panel Size X"=w252, "Panel size Y"=w251) -> (w242:cluster{"Panel Size X":dbl, "Panel size Y":dbl})  [unwired: 1 in]
            n27 = Unbundle By Name(w224) -> ("Panel Params"=w239:T5, "Scan Params[]"=w245:T11[])
            n28 = call "Get Robot Scan Direction.vi"("Scan Params[]"=w245) -> ("Scan Params"=w244:T11)  [unwired: 9 in, 1 out]
            n29 = call "PCB list format to GUI.vi"("delete ref"=w238, "File Panal Params"=w239) -> ("GUI Panel & PCB Params"=w240:T24)  [unwired: 13 in]
            n30 = Unbundle By Name(w240) -> ("PCBs List"=w231:T26)
            n31 = Bundle By Name(cluster=w244, "Size of Scanning Area"=w242, "Scan Offset"=cluster{"x":dbl, "y":dbl} {"x"=0.0, "y"=0.0} ("Scan Params.Scan Offset"), "Slice Step in mm"=10.0 ("Scan Params.Slice Step in mm"), "Triggering Distance in mm"=0.02 ("Scan Params.Triggering Distance in um"), "Triggering Distance in um"=20.0 ("Scan Params.Triggering Distance in mm"), "Profile Resolution"=Profile_Resolution."20 um" ("Scan Params.Profile Resolution")) -> (w228:T11)
            n32 = property class="Arr"(reference=w230, "Value"=w231) -> ()  [unwired: 1 in, 2 out]
            n33 = call "scan area dialog.vi"("error in (no error)"=w243, "Dongle Fitted event Refnum in"=w221, "Initial scanning area"=w242) -> ("error out"=w235:errorcluster, "Dongle fitted"=w217:bool, "Back"=w226:bool, "Scanning Area"=w241:T27)  [unwired: 5 in]
            n34 = property class="Clust (strict)"(reference=w229, "Value"=w228) -> (reference out=w227:refnum<vi>)  [unwired: 1 in, 1 out]
            n35 = case shown="True" w226 {
              tunnel: w241 -> [w261 _]
              tunnel: w227 -> [w254 _]
              tunnel: w228 -> [w260 _]
              tunnel: w224 -> [w256 w262]
              tunnel: [w255 w262] -> w232
              frame False {
                n36 = Bundle By Name(cluster=w260, "Size of Scanning Area"=w261) -> (w257:T11)
                n37 = property class="Clust (strict)"(reference=w254, "Value"=w257) -> ()  [unwired: 1 in, 2 out]
                n38 = call "Set Robot Scan Direction.vi"("Scan Direction"=enum32{"X", "Y", "X and Y"}."X" ("Robot Scan Direction"), "Scan Params"=w257) -> ("Scan Params"=w259:T11[])  [unwired: 9 in]
                n39 = Bundle By Name(cluster=w256, "Scan Params[]"=w259) -> (w255:T10)
              }
              frame True {
              }
            }
            n40 = Select(t=Import_ODB_state."Select PCBs", s=w226, f=Import_ODB_state."Select Fiducials") -> (s? t:f=w220:T16)
            n41 = Select(t=w220, s=w217, f=Import_ODB_state."Exit") -> (s? t:f=w218:T16)
          }
          frame "Select Fiducials" {
            n42 = Unbundle By Name(w269) -> ("Programming Files.IPF temp folder"=w288:path, "PCB Side"=w283:enum16{"Top", "Bottom"})
            n43 = Strip Path(path=w288) -> (stripped path=w287:path)  [unwired: 1 out]
            n44 = Strip Path(path=w287) -> (stripped path=w289:path)  [unwired: 1 out]
            n45 = Build Path(base path=w289, name or relative path="Extracted ODB") -> (appended path=w274:path)
            n46 = Bundle By Name(cluster=T19 {"Programming Files"={"PCB Design Identity"="", "ODB++ file"=path "", "Result  folder"=path "", "Tar file"=path ""}, "ODB file Converted?"=FALSE, "Inspection Setup Data"={"Inspection Program  file "=path "", "PCB Scanning Area"={"X"=0.0, " Y"=0.0}, "PCB Offset"={" X"=0.0, " Y"=0.0}, "Scanning area  bot left and top right"=[], "Fiducials from scan"=[], "TCF  file "=path "", "Robot Scan Params DBL"={"Zero"={"X"=0.0, "Y"=0.0}, "Zero Speed"={"X"=0.0, "Y"=0.0}, "Distance"={"X"=0.0, "Y"=0.0}, "Speed"={"X"=0.0, "Y"=0.0}, "# of Slices"=0.0, "Trigg Distance"=0.0, "Robot Scan Direction"=enum."X", "Next"={"Next Zero"={"X"=0.0, "Y"=0.0}, "Next Robot Scan Direction"=enum."X"}}, "Scan offset adjustment"={"X"=0.0, " Y"=0.0}}, "Panel Params"={"Name"="", "Pos & Rot"={"X"=0.0, "Y"=0.0, "Z"=0.0, "rotation"=0.0}, "PCBs List"=[], "PCB BarCode Params"=[], "Scan Type"=FALSE}, "PCB Outline File"=path "", "Inspection setup completed"=FALSE, "PCB Layer scanned"=enum."Bottom PCB Layer", "PCBs on a carrier"=FALSE, "Carrier Size"={"X"=0.0, "Y"=0.0}} ("Programming Data In"), "Programming Files.Result  folder"=w274) -> (w284:T19)
            n47 = call "Get CAD fiducials.vi"("Programming Data In"=w284, "Dongle Fitted event Refnum in"=w264, "APG"=TRUE, "Initial PCB Side"=w283, "error in (no error)"=w273) -> ("Dongle fitted"=w263:bool, "Inspection Data"=w281:T14, "Cancel"=w278:bool, "Back"=w271:bool, "error out"=w270:errorcluster)  [unwired: 6 in, 4 out]
            n48 = case shown="False" w263 {
              tunnel: [Import_ODB_state."Exit" w306] -> w282
              tunnel: w281 -> [_ w305]
              tunnel: w280 -> [_ w304]
              tunnel: w279 -> [_ w303]
              tunnel: w278 -> [_ w302]
              tunnel: [w291 w301] -> w277
              tunnel: w276 -> [_ w300]
              tunnel: w272 -> [w291 w299]
              tunnel: w271 -> [_ w298]
              tunnel: w270 -> [w292 w297]
              tunnel: w269 -> [_ w296]
              tunnel: w268 -> [_ w295]
              tunnel: [w292 w294] -> w267
              frame False {
              }
              frame True {
                n49 = case shown="False" w298 {
                  tunnel: [w318 Import_ODB_state."Scan area"] -> w306
                  tunnel: w305 -> [w316 _]
                  tunnel: w304 -> [w315 _]
                  tunnel: w303 -> [w313 _]
                  tunnel: w302 -> [w312 _]
                  tunnel: [w310 w333] -> w301
                  tunnel: w300 -> [w309 w323]
                  tunnel: w299 -> [w308 w333]
                  tunnel: w297 -> [w307 w331]
                  tunnel: [w307 w322] -> w294
                  tunnel: w296 -> [_ w328]
                  tunnel: w295 -> [_ w321]
                  frame False {
                    n50 = call "Reorder Fiducials.vi"("Inspection Data in"=w316) -> ("Inspection Data out"=w317:T14)  [unwired: 14 in]
                    n51 = call "inspection data format to GUI.vi"("delete"=w313, "Inspection Data"=w317) -> ("Fiducial List"=w314:T28)  [unwired: 13 in]
                    n52 = Bundle By Name(cluster=w308, "Inspection Data"=w317) -> (w311:T10)
                    n53 = property class="Arr"(reference=w315, "Value"=w314) -> ()  [unwired: 1 in, 2 out]
                    n54 = Select(t=w309, s=w312, f=w311) -> (s? t:f=w310:T10)
                    n55 = Select(t=Import_ODB_state."Cancel", s=w312, f=Import_ODB_state."Update CAD Picture") -> (s? t:f=w318:T16)
                  }
                  frame True {
                    n56 = call "Get Scan area.vi"("Inspection data"=w323, "error in (no error)"=w331, "Programming Data"=w328) -> ("error out"=w322:errorcluster, "Panel size Y"=w329:dbl, "Panel Size X"=w330:dbl)  [unwired: 6 in]
                    n57 = Bundle("Panel Size X"=w330, "Panel size Y"=w329) -> (w327:cluster{"Panel Size X":dbl, "Panel size Y":dbl})  [unwired: 1 in]
                    n58 = Unbundle By Name(w323) -> ("Scan Params[]"=w324:T11[])
                    n59 = call "Get Robot Scan Direction.vi"("Scan Params[]"=w324) -> ("Scan Params"=w325:T11)  [unwired: 9 in, 1 out]
                    n60 = Bundle By Name(cluster=w325, "Size of Scanning Area"=w327) -> (w326:T11)
                    n61 = property class="Clust (strict)"(reference=w321, "Value"=w326) -> ()  [unwired: 1 in, 2 out]
                  }
                }
              }
            }
          }
          frame "Update CAD Picture" {
            n62 = Unbundle By Name(w346) -> ("Board Library.Panel Picture File"=w336:path)
            n63 = Empty String/Path?(string/path=w336) -> (empty?=w350:bool)
            n64 = call-poly <userlib>:"File Exists__ogtk.vi"("file path"=w336) -> ("exists"=w351:bool)  [unwired: 6 in, 1 out]
            n65 = Compound Arithmetic op=AND(w351, invert w350) -> (w339:bool)
            n66 = Select(t=w336, s=w339, f=path "C:/a3Di" ("start path")) -> (s? t:f=w337:path)
            n67 = Strip Path(path=w336) -> (name=w335:string)  [unwired: 1 out]
            n68 = call "File Dialog"("start path"=w337, "prompt"="Select Panel Picture File", "default name"=w335, "error in"=w359, "pattern (all files)"="*.jpg;*.jpeg;*.jpe") -> ("selected path"=w348:path, "exists"=w342:bool, "cancelled"=w343:bool, "error out"=w347:errorcluster)  [unwired: 7 in]
            n69 = Compound Arithmetic op=AND(w342, invert w343) -> (w349:bool)
            n70 = case shown="True" w349 {
              tunnel: w357 -> [w366 w372]
              tunnel: [w366 w371] -> w356
              tunnel: w348 -> [_ w368]
              tunnel: w347 -> [w364 w370]
              tunnel: [w363 w370] -> w358
              tunnel: [path "" w368] -> w344
              tunnel: [Picture_FGV_commands."No Action" ("Panel Picture Command") Picture_FGV_commands."Set Update Picture" ("Panel Picture Command")] -> w352
              frame False {
                n71 = call <vilib>:"Clear Errors.vi"("error in (no error)"=w364) -> ("error out"=w363:errorcluster)  [unwired: 6 in]
              }
              frame True {
                n72 = Strip Path(path=w368) -> (name=w369:string)  [unwired: 1 out]
                n73 = Bundle By Name(cluster=w372, "CAD Picture File"=w369) -> (w371:T10)
              }
            }
            n74 = call "Panel Picture FGV.vi"("Panel Picture Command"=w352, "Panel Picture path in"=w344) -> ()  [unwired: 12 in, 2 out]
            n75 = Bundle By Name(cluster=w346, "Board Library.Panel Picture File"=w344) -> (w345:T3)
          }
          frame "Update TCF, save Files" {
            n76 = Unbundle By Name(w386) -> ("Programming Files.IPF temp folder"=w395:path, "PCB Side"=w407:enum16{"Top", "Bottom"})
            n77 = call "Inspection Program Write.vi"("error in (no error)"=w409, "IPF Folder"=w395, "data in"=w402) -> ("error out"=w408:errorcluster)  [unwired: 7 in, 1 out]
            n78 = Build Array(file_types."TCF" ("Descriptions"), file_types."CAD Outline" ("element"), file_types."CAD Labels" ("Descriptions"), file_types."CAD Pads" ("Descriptions"), file_types."CAD_Assembly" ("element")) -> (w400:T21[])
            n79 = for {
              tunnel: w400 -> [w546] mode=indexing
              tunnel: w408 -> [w545]
              tunnel: [w544] -> w401
              tunnel: [w543] -> w403 mode=indexing
              tunnel: w407 -> [w542]
              tunnel: w395 -> [w541]
              tunnel: w393 -> [w540]
              tunnel: w382 -> [w539]
              n80 = call "Extracted CAD to temp folder.vi"("Descriptions"=w546, "error in (no error)"=w545, "Assembly"=w539, "Extracted ODB"=w540, "IPF temp folder"=w541, "PCB Side"=w542) -> ("Temp file path"=w543:path, "error out"=w544:errorcluster)  [unwired: 12 in]
            }
            n81 = call "TCF Update.vi"("Programming Data In"=w386, "ODB import"=TRUE, "Dongle Fitted event Refnum in"=w375, "APG Config"=w384, "error in (no error)"=w401) -> ("Programming Data Out"=w405:T4, "Back"=w391:bool, "Dongle fitted"=w374:bool, "APG Config"=w380:T3, "error out"=w404:errorcluster)  [unwired: 6 in]
            n82 = case shown="True" w374 {
              tunnel: w405 -> [_ w448]
              tunnel: w404 -> [w418 w447]
              tunnel: w403 -> [_ w446]
              tunnel: w402 -> [w417 w445]
              tunnel: w400 -> [_ w444]
              tunnel: [w418 w443] -> w399
              tunnel: [w417 w442] -> w398
              tunnel: w397 -> [_ w441]
              tunnel: w396 -> [_ w440]
              tunnel: [Import_ODB_state."Exit" w439] -> w394
              tunnel: w393 -> [w419 w438]
              tunnel: [w419 w437] -> w392
              tunnel: w391 -> [_ w436]
              tunnel: [w415 w435] -> w390
              tunnel: w389 -> [_ w434]
              tunnel: w388 -> [_ w433]
              tunnel: w387 -> [_ w432]
              tunnel: w386 -> [w415 w431]
              tunnel: w384 -> [w414 w430]
              tunnel: [w416 w429] -> w383
              tunnel: w382 -> [w416 w428]
              tunnel: w381 -> [_ w427]
              tunnel: w380 -> [_ w426]
              tunnel: [w414 w425] -> w379
              tunnel: w378 -> [_ w424]
              tunnel: w376 -> [_ w423]
              tunnel: [FALSE TRUE] -> w373
              frame False {
              }
              frame True {
                n83 = case shown="False" w436 {
                  tunnel: w448 -> [w502 w535]
                  tunnel: w447 -> [w500 w536]
                  tunnel: w446 -> [w492 _]
                  tunnel: w445 -> [w491 w529]
                  tunnel: w444 -> [w490 _]
                  tunnel: [w489 w536] -> w443
                  tunnel: [w488 w530] -> w442
                  tunnel: w441 -> [w486 _]
                  tunnel: w440 -> [w482 _]
                  tunnel: w427 -> [w485 _]
                  tunnel: [Import_ODB_state."Exit" Import_ODB_state."Select Fiducials"] -> w439
                  tunnel: w438 -> [w483 w538]
                  tunnel: [w483 w538] -> w437
                  tunnel: [w461 w535] -> w435
                  tunnel: w434 -> [_ w534]
                  tunnel: w433 -> [_ w532]
                  tunnel: w432 -> [_ w531]
                  tunnel: w431 -> [w478 _]
                  tunnel: w430 -> [w460 w524]
                  tunnel: [w467 w525] -> w429
                  tunnel: w428 -> [w467 w525]
                  tunnel: w426 -> [w458 _]
                  tunnel: [w458 w524] -> w425
                  tunnel: w424 -> [w454 _]
                  tunnel: w423 -> [w451 _]
                  frame False {
                    w449 = TRUE ("Visible")
                    w450 = T29."Enabled" ("Disabled")
                    w493 = TRUE  # Set Initial flag
                    # "Save files to IPF"
                    n84 = Index Array(array=w492) -> (element #1=w496:path, element #2=w495:path)  [unwired: 2 in]
                    n85 = call-poly <vilib>:"Set Cursor.vi"("error in (no error)"=w500, "VI reference (current VI)"=w485, "icon"=u16 2) -> ("error out"=w501:errorcluster)  [unwired: 7 in, 1 out]
                    n86 = Unbundle By Name(w460) -> ("IPF Folder"=w479:path)
                    n87 = Unbundle By Name(w478) -> ("Programming Files.IPF temp folder"=w477:path)
                    n88 = call "APG Version.vi"() -> ("Versions"=w474:T30)  [unwired: 15 in]
                    n89 = Bundle By Name(cluster=w491, "Control File Relative Path"=w496, "PCB Outline File"=w495) -> (w462:T10)
                    n90 = Build Array (concatenate)(w490, file_types."ODB" ("Descriptions")) -> (w498:T21[])
                    n91 = Unbundle(w474) -> ("APG"=w473:cluster{"APG SIN":string, "APG version":string}, "Installed Programs"=w472:T31)
                    n92 = Strip Path(path=w477) -> (name=w476:string)  [unwired: 1 out]
                    n93 = Bundle("Program"=enum16{"APG", "Inspection Station"}."APG", "APG"=w473, "Installed Programs"=w472) -> (w475:T32)  [unwired: 1 in]
                    n94 = Build Path(base path=w479, name or relative path=w476) -> (appended path=w469:path)
                    n95 = call "Pack files.vi"("File type[]"=w498, "Programming Data In"=w502, "TCF/CAD Picture file"=w496, "APG Config"=w460, "error in (no error)"=w501) -> ("error out"=w481:errorcluster)  [unwired: 9 in, 1 out]
                    n96 = call-poly <userlib>:"Convert File Extension__ogtk.vi"("new ending (none)"="tar", "file name"=w469) -> ("new filename"=w468:path)  [unwired: 1 out]
                    n97 = call "Set Version.vi"("Inspection Prog File"=w468, "Versions"=w475, "error in (no error)"=w481) -> ("error out"=w480:errorcluster)  [unwired: 12 in]
                    n98 = call "Save inspection prog  to IPF.vi"("Programming Data in"=w502, "Set Initial flag"=w493, "APG Config"=w460, "data in"=w462, "error in"=w480) -> ("Programming Data out"=w461:T4, "data out"=w488:T10, "error out"=w465:errorcluster)  [unwired: 8 in]
                    n99 = call "Panel Picture FGV.vi"("Panel Picture Command"=Picture_FGV_commands."Get Picture action") -> ("Action"=w464:T33, "Panel Picture path out"=w463:path)  [unwired: 13 in]
                    n100 = case shown="\"Delete Picture\"" w464 {
                      tunnel: w465 -> [w507 w520 w523]
                      tunnel: w463 -> [w504 _ _]
                      tunnel: [w506 w511 w523] -> w456
                      tunnel: w461 -> [w505 w515 _]
                      tunnel: w460 -> [w503 w514 _]
                      frame "Update Picture" {
                        n101 = Build Array(file_types."CAD Picture" ("Descriptions")) -> (w508:T21[])
                        n102 = call "Pack files.vi"("File type[]"=w508, "Programming Data In"=w505, "TCF/CAD Picture file"=w504, "APG Config"=w503, "error in (no error)"=w507) -> ("error out"=w506:errorcluster)  [unwired: 9 in, 1 out]
                      }
                      frame "Delete Picture" {
                        n103 = Unbundle By Name(w514) -> ("IPF Folder"=w513:path)
                        n104 = Unbundle By Name(w515) -> ("Programming Files.IPF temp folder"=w519:path)
                        n105 = Strip Path(path=w519) -> (name=w518:string)  [unwired: 1 out]
                        n106 = Build Path(base path=w513, name or relative path=w518) -> (appended path=w517:path)
                        n107 = Build Array(file_types."CAD Picture" ("Descriptions")) -> (w521:T21[])
                        n108 = call-poly <userlib>:"Convert File Extension__ogtk.vi"("new ending (none)"="tar", "file name"=w517) -> ("new filename"=w510:path)  [unwired: 1 out]
                        n109 = call "Delete files.vi"("error in (no error)"=w520, "File type[]"=w521, "a3Di  tar file"=w510) -> ("error out"=w512:errorcluster)  [unwired: 7 in, 1 out]
                        n110 = call "clean tar.vi"("tar file"=w510, "error in (no error)"=w512) -> ("error out"=w511:errorcluster)  [unwired: 12 in, 1 out]
                      }
                      frame "No Action" {
                      }
                    }
                    n111 = call "Write apg_config.vi"("APG Config"=w458, "error in (no error)"=w456) -> ("APG Config out"=w459:T3, "error out"=w457:errorcluster)  [unwired: 12 in]
                    n112 = global write "apg_cfg_global.vi" "APG Config"(w459) -> ()
                    n113 = property on="Property Node" class="Bool"(reference=w486, error in=w457, "Visible"=w449, "DisabledEnum"=w450) -> (error out=w487:errorcluster)  [unwired: 1 out]
                    n114 = property on="Property Node" class="Bool"(reference=w482, error in=w487, "Visible"=w449, "DisabledEnum"=w450) -> (error out=w455:errorcluster)  [unwired: 1 out]
                    n115 = property on="Property Node" class="Bool"(reference=w454, error in=w455, "Visible"=w449, "DisabledEnum"=w450) -> (error out=w453:errorcluster)  [unwired: 1 out]
                    n116 = property on="Property Node" class="Bool"(reference=w451, error in=w453, "Visible"=w449, "DisabledEnum"=w450) -> (error out=w452:errorcluster)  [unwired: 1 out]
                    n117 = call-poly <vilib>:"Set Cursor.vi"("error in (no error)"=w452, "VI reference (current VI)"=w485, "icon"=u16 1) -> ("error out"=w489:errorcluster)  [unwired: 7 in, 1 out]
                  }
                  frame True {
                    # "Back to fiducial selection"
                    n118 = Unbundle By Name(w534) -> ("Inspection Data.Fiducial List"=w528:T34)
                    n119 = Bundle By Name(cluster=T14 {"Fiducial List"=[]} ("Inspection Data in"), "Fiducial List"=w528) -> (w526:T14)
                    n120 = call "inspection data format to GUI.vi"("delete"=w531, "Inspection Data"=w526) -> ("Fiducial List"=w533:T28)  [unwired: 13 in]
                    n121 = property class="Arr"(reference=w532, "Value"=w533) -> ()  [unwired: 1 in, 2 out]
                    n122 = Bundle By Name(cluster=w529, "Inspection Data"=w526) -> (w530:T10)
                  }
                }
              }
            }
          }
          frame "Cancel" {
            n123 = Unbundle By Name(w554) -> ("Programming Files.IPF temp folder"=w563:path)
            n124 = Build Array(file_types."Inspection Prog" ("IPF File"), file_types."TCF" ("IPF File")) -> (w560:T21[])
            n125 = call "Unpack files.vi"("IPF files[]"=w560, "APG Config"=w548, "IPF cmd"=IPF_cmd."Edit IPF", "Destination folder"=w563, "error in (no error)"=w557) -> ("error out"=w552:errorcluster)  [unwired: 10 in]
            n126 = One Button Dialog(message="ODB++ import cancelled") -> ()  [unwired: 1 in, 1 out]
          }
          frame "Exit" {
            n127 = call "Get IPF folder.vi"("error in (no error)"=w569) -> ("error out"=w568:errorcluster, "Results Folder"=w567:path)  [unwired: 5 in, 4 out]
            n128 = Bundle By Name(cluster=w566, "Programming Files.Result temp  folder"=w567) -> (w565:T4)
          }
        }
      }
    }
  }
  "error out" <- w20
  "Data out" <- w19
  "Programming Data out" <- w18
  "APG Config" <- w14
  "Dongle fitted" <- w1
